vi "Get Entry by ID.vi"(10 "ID":string, 11 "Object Dictionary in":refnum<class "Object Dictionary.lvclass">) -> (2 "Object Entry out":refnum<class "Object Entry.lvclass">, 3 "Object Dictionary out":refnum<class "Object Dictionary.lvclass">)   [LabVIEW 2024, in "EDS.lvlib" / "Object Dictionary.lvclass"]
uses:
  Object Dictionary.lvclass
  Object Entry/Object Entry.lvclass
  Object Dictionary.lvclass/Object Dictionary.ctl
  Object Entry/Object Entry.lvclass/Object Entry.ctl
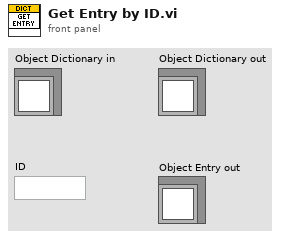
[diagram p1: front panel]
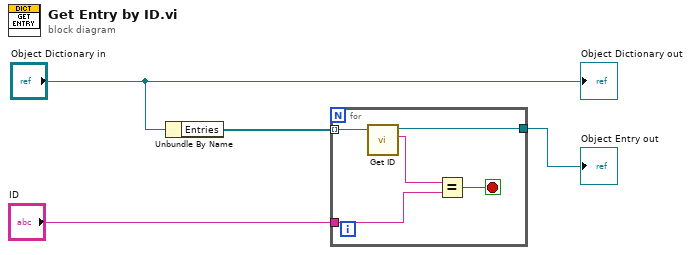
[diagram p0: block diagram]
diagram:
  n1 = Unbundle By Name("Object Dictionary in") -> ("Entries"=w3:refnum<class "Object Entry.lvclass">[])
  n2 = for {
    tunnel: w3 -> [w9] mode=indexing
    tunnel: "ID" -> [w7]
    tunnel: [w5] -> w1
    stop <- w6 stop-if-true
    n3 = call "Get ID.vi"("Object Entry in"=w9) -> ("ID"=w8:string, "Object Entry out"=w5:refnum<class "Object Entry.lvclass">)  [unwired: 8 in, 1 out]
    n4 = Equal?(x=w8, y=w7) -> (x = y?=w6:bool)
  }
  "Object Entry out" <- w1
  "Object Dictionary out" <- "Object Dictionary in"
